vi "PowerMeter.vi"() -> ()   [LabVIEW 2017]
uses:
  PowerMeter_Measurement.vi
panel:
  in  "instrument handle":refnum<visa-resource-name>="COM1"
  out "Active":bool
  out "Power Value":dbl caption="Optical Power [W]" format="%#_4p"
  in  "stop":bool
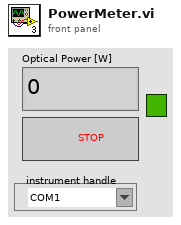
[diagram p1: front panel]
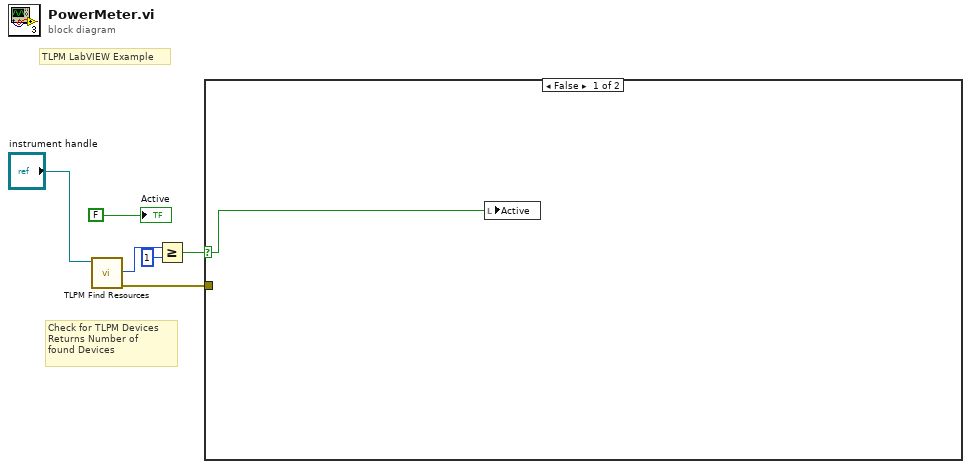
[diagram p0: block diagram]
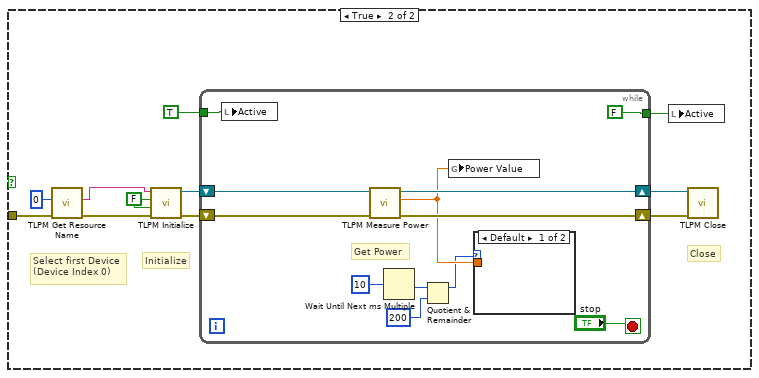
[diagram p2: hidden frame]
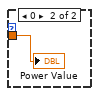
[diagram p3: hidden frame]
diagram:
  # "TLPM LabVIEW Example"
  # "Check for TLPM Devices\nReturns Number of\nfound Devices"
  n1 = call "TLPM Find Resources.vi"("instrument handle"="instrument handle") -> ("error out"=w5:errorcluster, "Resource Count"=w3:u32)  [unwired: 8 in, 1 out]
  n2 = Greater Or Equal?(x=w3, y=u32 1) -> (x >= y?=w4:bool)
  n3 = case shown="False" w4 {
    selector: w4 -> [w7 _]
    tunnel: w5 -> [_ w15]
    frame False {
      n4 = local write "Active"(w7) -> ()
    }
    frame True {
      w13 = FALSE ("ID Query (Do Query)")
      # "Close"
      # "Initialize"
      # "Select first Device\n(Device Index 0)"
      n5 = call "TLPM Get Resource Name.vi"("error in (no error)"=w15, "Index (0)"=u32 0 ("Device Index")) -> ("error out"=w17:errorcluster, "Resource Name"=w8:string)  [unwired: 7 in, 1 out]
      n6 = call "TLPM Initialize.vi"("error in (no error)"=w17, "Reset Device (Reset Device)"=w13, "ID Query (Do Query)"=w13, "resource name"=w8) -> ("error out"=w11:errorcluster, "instrument handle out"=w12:refnum<visa-resource-name>)  [unwired: 6 in]
      n7 = while {
        shift-right: [w25] -> w18
        shift-left: w12 -> [w30]
        shift-right: [w24] -> w16
        shift-left: w11 -> [w29]
        tunnel: [FALSE ("Active")] -> w10
        tunnel: TRUE ("Active") -> [w26]
        stop <- "stop" stop-if-true
        # "Get Power"
        n8 = local write "Active"(w26) -> ()
        n9 = call "TLPM Measure Power.vi"("error in (no error)"=w29, "instrument handle"=w30) -> ("error out"=w24:errorcluster, "Power"=w23:dbl, "instrument handle out"=w25:refnum<visa-resource-name>)  [unwired: 7 in]
        n10 = Wait Until Next ms Multiple(millisecond multiple=u32 10 ("milliseconds to wait")) -> (millisecond timer value=w21:u32)
        n11 = Quotient & Remainder(x=w21, y=u32 200) -> (x-y*floor(x/y)=w19:u32)  [unwired: 1 out]
        n12 = global write "PowerMeter_Measurement.vi" "Power Value"(w23) -> ()
        n13 = case shown="Default" w19 {
          tunnel: w23 -> [_ w31]
          frame Default {
          }
          frame 0 {
            "Power Value" <- w31
          }
        }
      }
      n14 = local write "Active"(w10) -> ()
      n15 = call "TLPM Close.vi"("error in (no error)"=w16, "instrument handle"=w18) -> ()  [unwired: 9 in, 1 out]
    }
  }
  "Active" <- FALSE ("Active")
